vi "TagBus_Write Table from Cluster (DVR).vi"(7 "Clust Refnum":refnum<vi>, 10 "Index Array":i32[](array[numeric]), 11 "Data Value Reference in":refnum<data-value>) -> (3 "Data Value Reference out":refnum<data-value>)   [LabVIEW 2015, in "TagBus.lvclass"]
uses:
  TagBus.lvclass
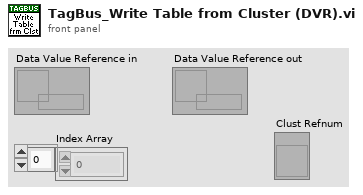
[diagram p1: front panel]
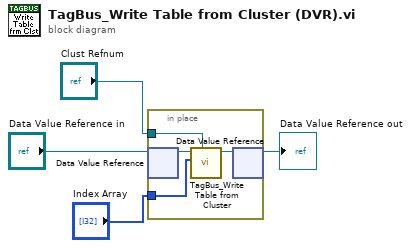
[diagram p0: block diagram]
diagram:
  n1 = in-place {
    in-place-border: "Index Array" -> [w6]
    in-place-border: "Clust Refnum" -> [w7]
    n2 = in-place-dvr #1("Data Value Reference in") -> (w8:refnum<class "TagBus.lvclass">)  [unwired: 1 out]
    n3 = call "TagBus_Write Table from Cluster.vi"("Clust Refnum"=w7, "Index Array"=w6, "TagBus in"=w8) -> ("TagBus out"=w5:refnum<class "TagBus.lvclass">)  [unwired: 8 in]
    n4 = in-place-dvr #1(w5) -> (→"Data Value Reference out":refnum<data-value>)  [unwired: 1 out]
  }
